vi "Configuration.Get Settings.vi"(11 "Configuration in":refnum<class "Configuration.lvclass">) -> (2 "settings":T1, 3 "Configuration out":refnum<class "Configuration.lvclass">)   [LabVIEW 2017, in "DSF Core.lvlib" / "Configuration.lvclass"]
uses:
  Configuration.lvclass
  DSF Configuration API/Public/Controls/DSF Settings Info.ctl
  Configuration.lvclass/Configuration.ctl
  DSF Core.lvlib
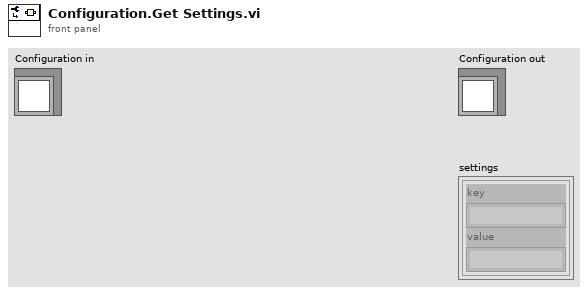
[diagram p1: front panel]
types:
  T1 = typedef "DSF Core.lvlib/DSF Settings Info.ctl" = cluster{"key":string, "value":string}[]
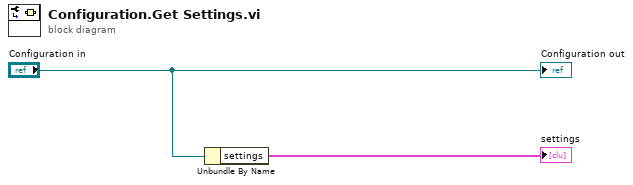
[diagram p0: block diagram]
diagram:
  n1 = Unbundle By Name("Configuration in") -> ("settings"=→"settings":T1)
  "Configuration out" <- "Configuration in"
